vi "Build Clear All String Request.vi"(9 "Time Stamp In":timestamp, 10 "Names Array In":string[](array[string]), 11 "Parent NodeID In":string) -> (2 "Requests Array Out":T1[](array[typedef]) {"node status" items=["Good"=0, "Uncertain"=1073741824, "Uncertain_InitialValue"=1083310080, "Uncertain_LastUsableValue"=1083179008, "Uncertain_SensorNotAccurate"=1083375616, "Uncertain_EngineeringUnitsExceeded"=1083441152, "Bad"=2147483648, "Bad_NoCommunication"=2150694912, "Bad_NotReadable"=2151284736, "Bad_NotWritable"=2151350272, "Bad_OutOfRange"=2151415808, "Bad_WaitingForInitialData"=2150760448]})   [LabVIEW 2024]
uses:
  <vilib>/OPCUA/controls/NodeId.ctl
  <vilib>/OPCUA/controls/Write Status.ctl
  <vilib>/OPCUA/controls/Write Variant Request.ctl
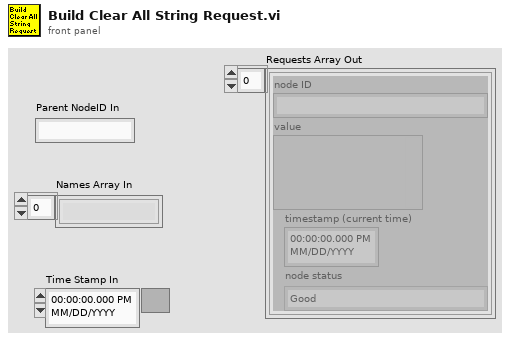
[diagram p1: front panel]
types:
  T1 = typedef "Write Variant Request.ctl" = cluster{"node ID":T2, "value":variant, "timestamp (current time)":timestamp, "node status":T3}
  T2 = typedef "NodeId.ctl" = string
  T3 = typedef "Write Status.ctl" = u32
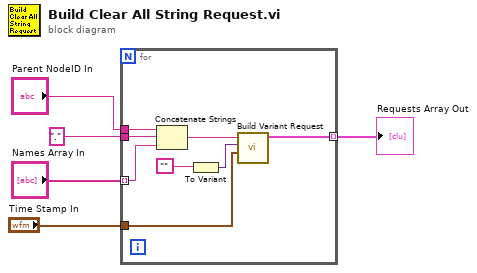
[diagram p0: block diagram]
diagram:
  n1 = for {
    tunnel: "." -> [w13]
    tunnel: "Parent NodeID In" -> [w12]
    tunnel: "Names Array In" -> [w11] mode=indexing
    tunnel: "Time Stamp In" -> [w7]
    tunnel: [w6] -> w1 mode=indexing
    n2 = Concatenate Strings(w12, w13, w11) -> (w10:string)
    n3 = To Variant(anything="") -> (Variant=w9:variant)
    n4 = call "Build Variant Request.vi"("Time Stamp In"=w7, "variant in"=w9, "Node ID In"=w10) -> ("request out"=w6:T1)  [unwired: 8 in]
  }
  "Requests Array Out" <- w1
